vi "read_buffer.vi"(0 "Buffer":string) -> (1 "Buffer Out":string, 2 "New Packet":bool, 3 "Data":u8[](array[numeric]))   [LabVIEW 2022 SP3]
uses:
  12d3c856-85df-4f50-943d-d50f2d9941f5.vi
  17ba3664-fc9c-437e-8621-ab08f704feab.vi
panel:
  in  "Sync End":u8=109
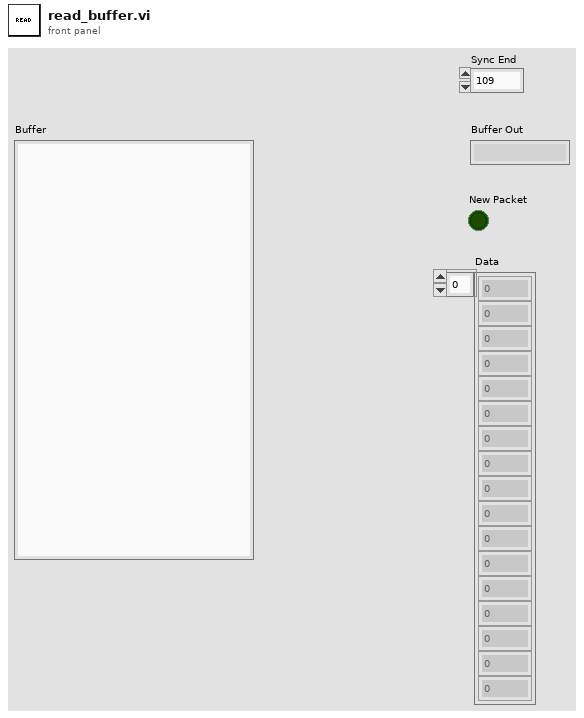
[diagram p1: front panel]
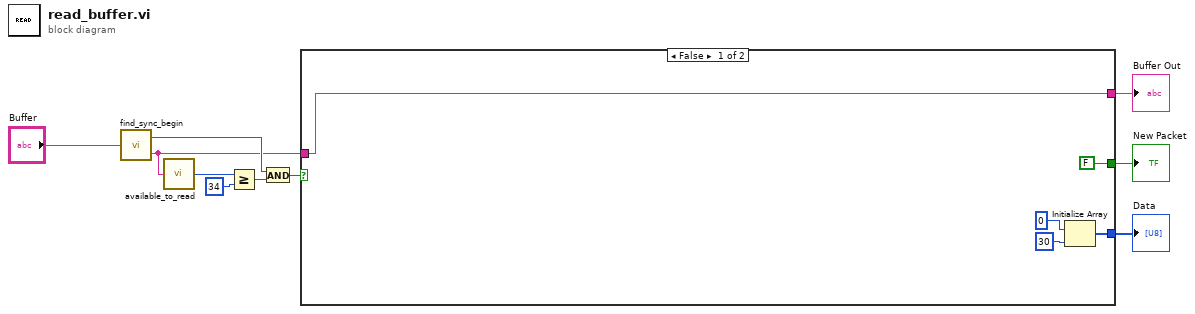
[diagram p0: block diagram]
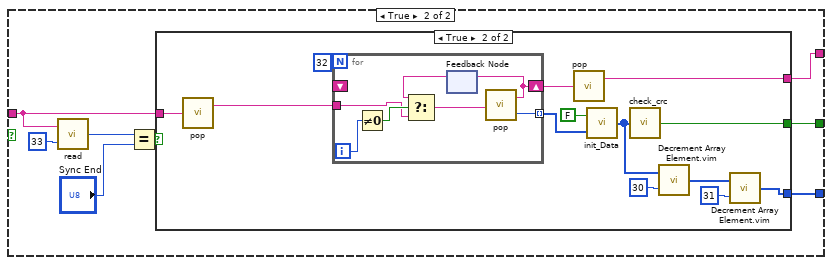
[diagram p2: hidden frame]
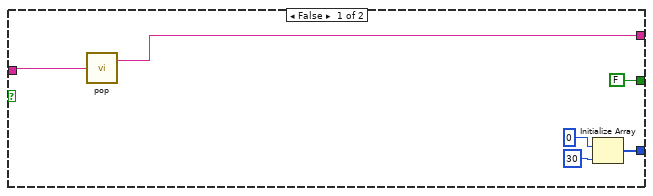
[diagram p3: hidden frame]
diagram:
  n1 = call "find_sync_begin.vi"("Buffer"="Buffer") -> ("Found"=w5:bool, "Buffer Out"=w3:string)
  n2 = call "available_to_read.vi"("Buffer"=w3) -> ("Available to read"=w9:u32)
  n3 = Greater Or Equal?(x=w9, y=u32 34) -> (x >= y?=w6:bool)
  n4 = And(x=w5, y=w6) -> (x .and. y?=w7:bool)
  n5 = case shown="False" w7 {
    tunnel: w3 -> [w15 w20]
    tunnel: [w15 w17] -> w4
    tunnel: [FALSE ("CRC check") w19] -> w2
    tunnel: [w11 w18] -> w1
    frame False {
      n6 = Initialize Array(u8 0 ("element"), 30 ("dimension size")) -> (w11:u8[])
    }
    frame True {
      n7 = call "read.vi"("Index"=u16 33, "Buffer"=w20) -> ("Value"=w22:u8)
      n8 = Equal?(x=w22, y="Sync End") -> (x = y?=w21:bool)
      n9 = case shown="True" w21 {
        tunnel: w20 -> [w25 w42]
        tunnel: [FALSE ("CRC check") w36] -> w19
        tunnel: [w27 w31] -> w18
        tunnel: [w24 w30] -> w17
        frame False {
          n10 = call "pop.vi"("Buffer"=w25) -> ("New Buffer"=w24:string)  [unwired: 1 out]
          n11 = Initialize Array(u8 0 ("element"), 30 ("dimension size")) -> (w27:u8[])
        }
        frame True {
          n12 = call "pop.vi"("Buffer"=w42) -> ("New Buffer"=w39:string)  [unwired: 1 out]
          n13 = for {
            N: 32 -> [_]
            tunnel: [w49] -> w40 mode=indexing
            tunnel: w39 -> [w46]
            shift-right: [w43] -> w38
            shift-left: _ -> [_]
            i -> [w47]
            n14 = Not Equal To 0?(x=w47) -> (x != 0?=w48:bool)
            n15 = feedback #1() -> (w44:string)  [unwired: 1 in]
            n16 = Select(t=w44, s=w48, f=w46) -> (s? t:f=w45:string)
            n17 = call "pop.vi"("Buffer"=w45) -> ("New Buffer"=w43:string, "Value"=w49:u8)
            n18 = feedback-in #1(w43) -> ()
          }
          n19 = call "pop.vi"("Buffer"=w38) -> ("New Buffer"=w30:string)  [unwired: 1 out]
          n20 = call "init_Data.vi"("Input"=w40, "Zerar CRC"=FALSE) -> ("Output"=w33:u8[])
          n21 = call "check_crc.vi"("Data"=w33) -> ("CRC check"=w36:bool)
          n22 = call "Decrement Array Element.vim"("index"=30, "array in"=w33) -> ("array out"=w32:u8[])
          n23 = call "Decrement Array Element.vim"("index"=31, "array in"=w32) -> ("array out"=w31:u8[])
        }
      }
    }
  }
  "Buffer Out" <- w4
  "Data" <- w1
  "New Packet" <- w2
